vi "RobotStatusFGV.vi"(0 "Application Interface in":refnum<class "Application Interface.lvclass">, 1 "Robot Status in":T1, 5 "error in (no error)":errorcluster, 9 "Action (Read)":T5=enum."Get Last Status") -> (14 "Application Interface out":refnum<class "Application Interface.lvclass">, 15 "Robot Status out":T1, 19 "error out":errorcluster)   [LabVIEW 2019, in "Application Interface.lvclass"]
uses:
  Application Interface.lvclass
  Robot/Universal Robot/RobotStatus.ctl
  Robot/Universal Robot/RobotMode.ctl
  Robot/Universal Robot/OperationalMode.ctl
  Robot/Universal Robot/SafetyStatus.ctl
  FGVAction.ctl
  Robot/Universal Robot/Universal Robot.lvclass
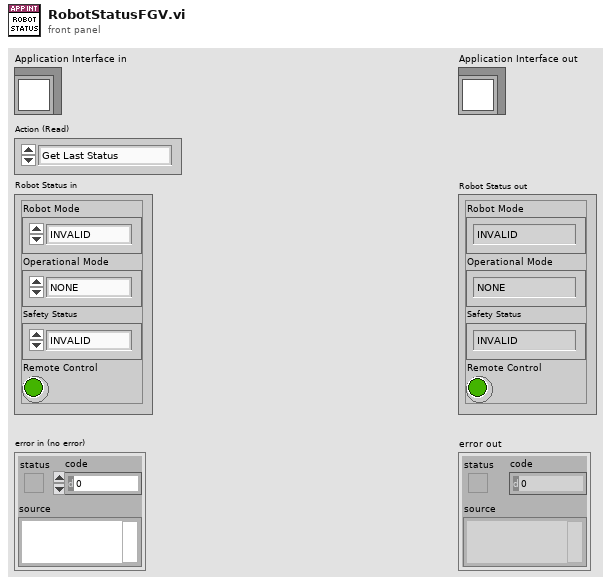
[diagram p1: front panel]
types:
  T1 = typedef "Universal Robot.lvclass/RobotStatus.ctl" = cluster{"Robot Mode":T2, "Operational Mode":T3, "Safety Status":T4, "Remote Control":bool}
  T2 = typedef "Universal Robot.lvclass/RobotMode.ctl" = enum16{"INVALID", "NO_CONTROLLER", "DISCONNECTED", "CONFIRM_SAFETY", "BOOTING", "POWER_OFF", "POWER_ON", "IDLE", "BACKDRIVE", "RUNNING"}
  T3 = typedef "Universal Robot.lvclass/OperationalMode.ctl" = enum16{"NONE", "MANUAL", "AUTOMATIC"}
  T4 = typedef "Universal Robot.lvclass/SafetyStatus.ctl" = enum16{"INVALID", "NORMAL", "REDUCED", "PROTECTIVE_STOP", "RECOVERY", "SAFEGUARD_STOP", "SYSTEM_EMERGENCY_STOP", "ROBOT_EMERGENCY_STOP", "VIOLATION", "FAULT", "AUTOMATIC_MODE_SAFEGAURD_STOP", "SYSTEM_THREE_POSITION_ENABLING_STOP"}
  T5 = typedef "Application Interface.lvclass/FGVAction.ctl" = enum16{"Initialize", "Get Last Status", "Update Status"}
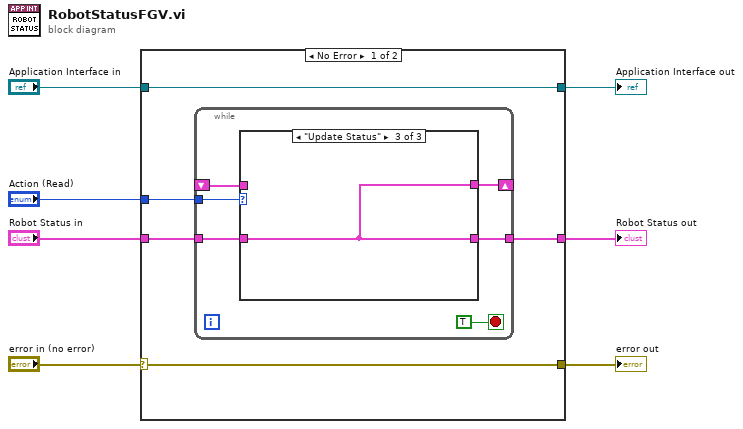
[diagram p0: block diagram]
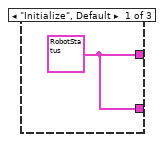
[diagram p2: hidden frame]
diagram:
  n1 = case shown="No Error" "error in (no error)" {
    selector: "error in (no error)" -> [w8 w23]
    tunnel: [w8 w23] -> w6
    tunnel: [w12 w22] -> w4
    tunnel: "Application Interface in" -> [w12 w22]
    tunnel: "Robot Status in" -> [w11 _]
    tunnel: "Action (Read)" -> [w10 _]
    tunnel: [w9 _] -> w1
    frame No Error {
      n2 = while {
        tunnel: w11 -> [w17]
        tunnel: w10 -> [w16]
        shift-right: [w15] -> _
        shift-left: _ -> [w14]
        tunnel: [w13] -> w9
        stop <- TRUE stop-if-true
        n3 = case shown="\"Update Status\"" w16 {
          tunnel: w17 -> [_ _ w21]
          tunnel: [w19 w20 w21] -> w15
          tunnel: w14 -> [_ w20 _]
          tunnel: [w19 w20 w21] -> w13
          frame "Initialize", Default {
            w19 = T1 {"Robot Mode"=enum."INVALID", "Operational Mode"=enum."NONE", "Safety Status"=enum."INVALID", "Remote Control"=FALSE} ("Robot Status in")
          }
          frame "Get Last Status" {
          }
          frame "Update Status" {
          }
        }
      }
    }
    frame Error {
    }
  }
  "error out" <- w6
  "Application Interface out" <- w4
  "Robot Status out" <- w1
